vi "Begin.vi"(8 "error in":errorcluster) -> (0 "error out":errorcluster)   [LabVIEW 2018]
doc: "Called before other user functions, this VI is expected to open initial I/O refnums, load in file data, and do all program initialization. Notice that the <B>error out</B> terminal is simply used for data flow. Wiring it to other structures or subVIs ensures that this VI runs first."
uses:
  <vilib>/Rock Robotics/SystemInterfaces/DIO/FPGA_DIOPWMChannel.ctl
  <vilib>/Rock Robotics/WPI/SafetyOutput/WPI_SafetyOutputConfigMenu.ctl
  <vilib>/Rock Robotics/WPI/DriverStation/WPI_DriverStationRobotMode2.ctl
  <vilib>/Rock Robotics/WPI/Joystick/WPI_JoystickDeviceEnum.ctl
  <vilib>/Rock Robotics/SystemInterfaces/AI/FPGA_AIChannel.ctl
  <vilib>/Rock Robotics/WPI/RobotDrive/WPI_RobotDriveOpen2MotorWithTalon.vi
  Robot Global Data.vi
  <vilib>/Rock Robotics/Network Tables/NT Write String Array.vi
  <vilib>/Rock Robotics/WPI/ThirdParty/Phoenix-LabVIEW/Pigeon IMU/CTRE_PigeonIMU_Open_TalonSRX.vi
  <vilib>/Rock Robotics/WPI/Solenoid/WPI_SolenoidOpenSingle.vi
panel:
  in  "error in 2":errorcluster
  out "error out 2":errorcluster
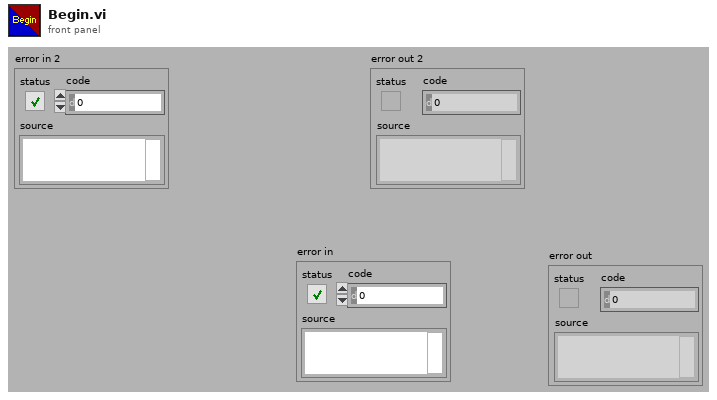
[diagram p1: front panel]
types:
  T1 = typedef "FPGA_AIChannel.ctl" = enum8{"AI 0", "AI 1", "AI 2", "AI 3", "AI MXP 0", "AI MXP 1", "AI MXP 2", "AI MXP 3", "Invalid"}
  T2 = typedef "WPI_JoystickDeviceEnum.ctl" = enum16{"USB 0", "USB 1", "USB 2", "USB 3", "USB 4", "USB 5"}
  T3 = typedef "WPI_DriverStationRobotMode2.ctl" = enum16{"Autonomous Disabled", "Autonomous Enabled", "Teleop Disabled", "Teleop Enabled", "Disconnected", "Finish", "Test Disabled", "Test Enabled", "Emergency Stopped"}
  T4 = typedef "WPI_SafetyOutputConfigMenu.ctl" = enum16{"Enable", "Disable"}
  T5 = typedef "FPGA_DIOPWMChannel.ctl" = enum8{"PWM 0", "PWM 1", "PWM 2", "PWM 3", "PWM 4", "PWM 5", "PWM 6", "PWM 7", "PWM 8", "PWM 9", "PWM MXP 0", "PWM MXP 1", "PWM MXP 2", "PWM MXP 3", "PWM MXP 4", "PWM MXP 5", "PWM MXP 6", "PWM MXP 7", "PWM MXP 8", "PWM MXP 9", "Invalid"}
  T6 = typedef "WPI_JoystickDevRef.ctl" = cluster{"Device":T2}
  T7 = typedef "WPI_RobotDriveDevRef.ctl" = cluster{"DevStatus":errorcluster, "Motors[]":T8[], "Square Inputs":bool, "Max Output":dbl}
  T8 = typedef "WPI_MotorControlDeviceRef.ctl" = cluster{"DeviceStatus":errorcluster, "Type":T9, "PWM":cluster{"PWM Channel":T5, "DeadBand":T10}, "CAN":cluster{"Device Number":u8, "SetOutput VI Ref":variant, "GetOutput VI Ref":variant, "Enable VI Ref":variant, "Disable VI Ref":variant, "Data":variant}, "Invert":bool, "DIO PWM":cluster{"PWM \"Enable\" Channel":T5, "DIOChannel":T11, "PWM Rate":dbl}}
  T9 = typedef "WPI_MotorControlType.ctl" = enum16{"PWM", "CAN", "DIO PWM"}
  T10 = typedef "WPI_PWMDeadband.ctl" = cluster{"Name":string, "maxPositivePwm":i32, "minPositivePwm":i32, "centerPwm":i32, "maxNegativePwm":i32, "minNegativePwm":i32, "angularRange":u16}
  T11 = typedef "FPGA_DIOChannel.ctl" = enum8{"DIO 0", "DIO 1", "DIO 2", "DIO 3", "DIO 4", "DIO 5", "DIO 6", "DIO 7", "DIO 8", "DIO 9", "DIO MXP 0", "DIO MXP 1", "DIO MXP 2", "DIO MXP 3", "DIO MXP 4", "DIO MXP 5", "DIO MXP 6", "DIO MXP 7", "DIO MXP 8", "DIO MXP 9", "DIO MXP 10", "DIO MXP 11", "DIO MXP 12", "DIO MXP 13", "DIO MXP 14", "DIO MXP 15", "SPI Port CS1", "SPI Port CS2", "SPI Port CS3", "SPI Port MISO", "SPI Port MOSI", "Invalid"}
  T12 = typedef "WPI_AnalogChannelDevRef.ctl" = cluster{"DevStatus":errorcluster, "Analog Channel":T1}
  T13 = typedef "CTRE_PigeonIMU_DeviceRef.ctl" = cluster{"DeviceStatus":errorcluster, "Device Number":u8, "Type":T14, "Device ID":u32, "Handle":u64, "UsageFrame":u32, "Library Path":path}
  T14 = typedef "CTRE_PigeonIMU_ConnectionType.ctl" = u32
  T15 = typedef "WPI_SolenoidDevRef.ctl" = cluster{"DevStatus":errorcluster, "Pneumatics Control Module":u8, "Forward Solenoid Channel":T16, "Reverse Solenoid Channel":T16}
  T16 = typedef "WPI_SolenoidChannel.ctl" = enum8{"Solenoid 0", "Solenoid 1", "Solenoid 2", "Solenoid 3", "Solenoid 4", "Solenoid 5", "Solenoid 6", "Solenoid 7", "Invalid"}
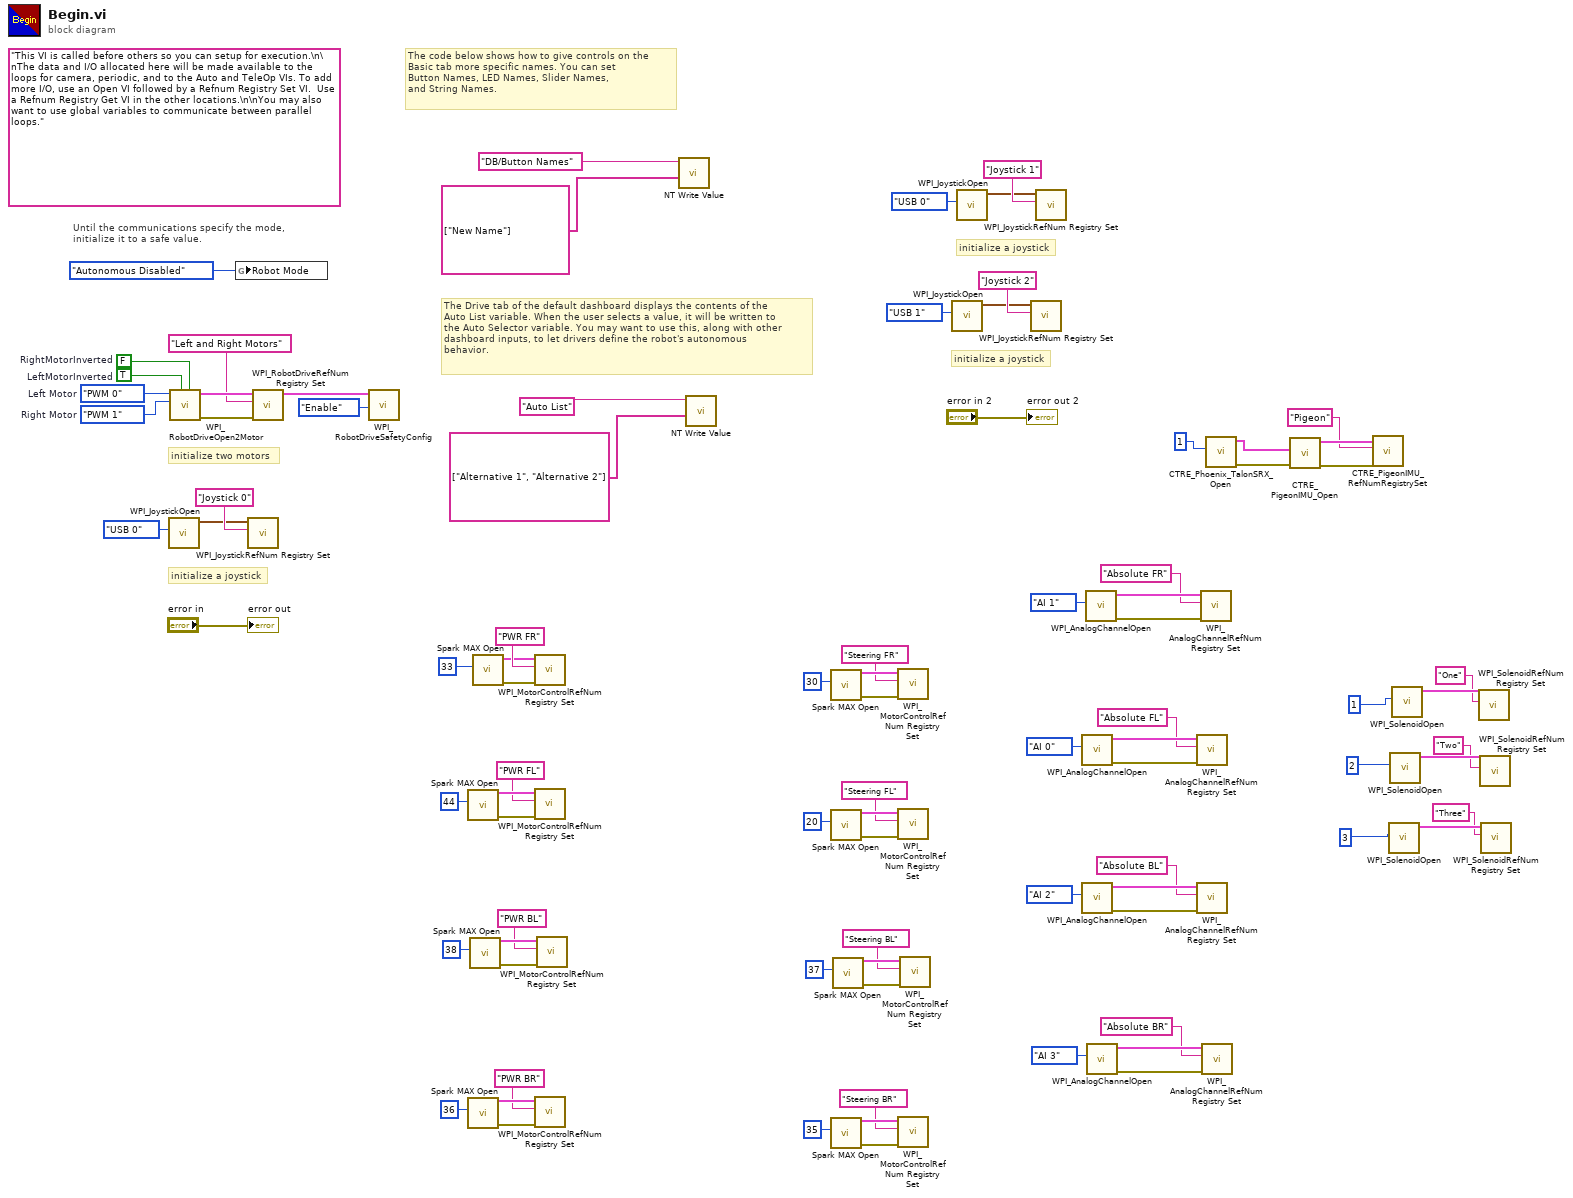
[diagram p0: block diagram]
diagram:
  (unwired) "This VI is called before others so you can setup for execution.\n\nThe data and I/O allocated here will be made available to the loops for camera, periodic, and to the Auto and TeleOp VIs. To add more I/O, use an Open VI followed by a Refnum Registry Set VI.  Use a Refnum Registry Get VI in the other locations.\n\nYou may also want to use global variables to communicate between parallel loops."
  w82 = FPGA_DIOPWMChannel."PWM 1"  # Right Motor
  w83 = FPGA_DIOPWMChannel."PWM 0"  # Left Motor
  w87 = TRUE  # LeftMotorInverted
  w88 = FALSE  # RightMotorInverted
  # "initialize a joystick"
  # "The Drive tab of the default dashboard displays the contents of the\nAuto List variable. When the user selects a value, it will be written to\nthe Auto Selector variable. You may want to use this, along with other\ndashboard inputs, to let drivers define the robot's autonomous\nbehavior."
  # "The code below shows how to give controls on the\nBasic tab more specific names. You can set\nButton Names, LED Names, Slider Names,\nand String Names."
  # "initialize a joystick"
  # "initialize a joystick"
  # "Until the communications specify the mode,\ninitialize it to a safe value."
  # "initialize two motors"
  n1 = call <vilib>:"WPI_JoystickOpen.vi"("JoystickDevice"=WPI_JoystickDeviceEnum."USB 0") -> ("JoystickDevRef"=w77:T6)  [unwired: 10 in]
  n2 = call-poly <vilib>:"WPI_RobotDriveOpen2Motor.vi"("Right Motor Inverted"=w88, "Left Motor Inverted"=w87, "Right Motor"=w82, "Left Motor"=w83) -> ("error out"=w84:errorcluster, "RobotDriveDevRef"=w86:T7)  [unwired: 1 in, 5 out]
  n3 = global write "Robot Global Data.vi" "Robot Mode"(WPI_DriverStationRobotMode2."Autonomous Disabled" ("Robot Mode")) -> ()
  n4 = call <vilib>:"WPI_JoystickRefNum Registry Set.vi"("refnum name"="Joystick 0", "JoystickDevRef"=w77) -> ()  [unwired: 8 in, 2 out]
  n5 = call <vilib>:"WPI_RobotDriveRefNum Registry Set.vi"("error in (no error)"=w84, "refnum name"="Left and Right Motors", "RobotDriveDevRef"=w86) -> ("RobotDriveDevRef"=w81:T7)  [unwired: 1 in, 7 out]
  n6 = call <vilib>:"WPI_RobotDriveSafetyConfig.vi"("mode"=WPI_SafetyOutputConfigMenu."Enable", "RobotDriveDevRef"=w81) -> ()  [unwired: 8 in, 2 out]
  n7 = call <vilib>:"Spark MAX Open.vi"("Device Number"=u8 44) -> ("error out"=w61:errorcluster, "MotorControlDeviceRef"=w62:T8)  [unwired: 9 in]
  n8 = call <vilib>:"Spark MAX Open.vi"("Device Number"=u8 36) -> ("error out"=w55:errorcluster, "MotorControlDeviceRef"=w56:T8)  [unwired: 9 in]
  n9 = call <vilib>:"Spark MAX Open.vi"("Device Number"=u8 38) -> ("error out"=w58:errorcluster, "MotorControlDeviceRef"=w59:T8)  [unwired: 9 in]
  n10 = call <vilib>:"Spark MAX Open.vi"("Device Number"=u8 33) -> ("error out"=w52:errorcluster, "MotorControlDeviceRef"=w53:T8)  [unwired: 9 in]
  n11 = call <vilib>:"WPI_MotorControlRefNum Registry Set.vi"("error in (no error)"=w52, "refnum name"="PWR FR", "MotorControlDevRef"=w53) -> ()  [unwired: 7 in, 2 out]
  n12 = call <vilib>:"WPI_MotorControlRefNum Registry Set.vi"("error in (no error)"=w61, "refnum name"="PWR FL", "MotorControlDevRef"=w62) -> ()  [unwired: 7 in, 2 out]
  n13 = call <vilib>:"WPI_MotorControlRefNum Registry Set.vi"("error in (no error)"=w55, "refnum name"="PWR BR", "MotorControlDevRef"=w56) -> ()  [unwired: 7 in, 2 out]
  n14 = call <vilib>:"WPI_MotorControlRefNum Registry Set.vi"("error in (no error)"=w58, "refnum name"="PWR BL", "MotorControlDevRef"=w59) -> ()  [unwired: 7 in, 2 out]
  n15 = call-poly <vilib>:"NT Write Value.vi"("String Array"=string[] ["New Name"], "Name"="DB/Button Names") -> ()  [unwired: 9 in, 1 out]
  n16 = call-poly <vilib>:"NT Write Value.vi"("String Array"=string[] ["Alternative 1", "Alternative 2"], "Name"="Auto List") -> ()  [unwired: 9 in, 1 out]
  n17 = call <vilib>:"Spark MAX Open.vi"("Device Number"=u8 30) -> ("error out"=w46:errorcluster, "MotorControlDeviceRef"=w47:T8)  [unwired: 9 in]
  n18 = call <vilib>:"Spark MAX Open.vi"("Device Number"=u8 20) -> ("error out"=w43:errorcluster, "MotorControlDeviceRef"=w44:T8)  [unwired: 9 in]
  n19 = call <vilib>:"Spark MAX Open.vi"("Device Number"=u8 35) -> ("error out"=w37:errorcluster, "MotorControlDeviceRef"=w38:T8)  [unwired: 9 in]
  n20 = call <vilib>:"Spark MAX Open.vi"("Device Number"=u8 37) -> ("error out"=w40:errorcluster, "MotorControlDeviceRef"=w41:T8)  [unwired: 9 in]
  n21 = call <vilib>:"WPI_MotorControlRefNum Registry Set.vi"("error in (no error)"=w46, "refnum name"="Steering FR", "MotorControlDevRef"=w47) -> ()  [unwired: 7 in, 2 out]
  n22 = call <vilib>:"WPI_MotorControlRefNum Registry Set.vi"("error in (no error)"=w43, "refnum name"="Steering FL", "MotorControlDevRef"=w44) -> ()  [unwired: 7 in, 2 out]
  n23 = call <vilib>:"WPI_MotorControlRefNum Registry Set.vi"("error in (no error)"=w37, "refnum name"="Steering BR", "MotorControlDevRef"=w38) -> ()  [unwired: 7 in, 2 out]
  n24 = call <vilib>:"WPI_MotorControlRefNum Registry Set.vi"("error in (no error)"=w40, "refnum name"="Steering BL", "MotorControlDevRef"=w41) -> ()  [unwired: 7 in, 2 out]
  n25 = call <vilib>:"WPI_JoystickOpen.vi"("JoystickDevice"=WPI_JoystickDeviceEnum."USB 1") -> ("JoystickDevRef"=w65:T6)  [unwired: 10 in]
  n26 = call <vilib>:"WPI_JoystickOpen.vi"("JoystickDevice"=WPI_JoystickDeviceEnum."USB 0") -> ("JoystickDevRef"=w73:T6)  [unwired: 10 in]
  n27 = call <vilib>:"WPI_JoystickRefNum Registry Set.vi"("refnum name"="Joystick 2", "JoystickDevRef"=w65) -> ()  [unwired: 8 in, 2 out]
  n28 = call <vilib>:"WPI_JoystickRefNum Registry Set.vi"("refnum name"="Joystick 1", "JoystickDevRef"=w73) -> ()  [unwired: 8 in, 2 out]
  n29 = call <vilib>:"WPI_AnalogChannelOpen.vi"("Analog Channel"=FPGA_AIChannel."AI 0") -> ("error out"=w28:errorcluster, "AIDeviceRef"=w27:T12)  [unwired: 9 in]
  n30 = call <vilib>:"WPI_AnalogChannelOpen.vi"("Analog Channel"=FPGA_AIChannel."AI 2") -> ("error out"=w25:errorcluster, "AIDeviceRef"=w24:T12)  [unwired: 9 in]
  n31 = call <vilib>:"WPI_AnalogChannelOpen.vi"("Analog Channel"=FPGA_AIChannel."AI 1") -> ("error out"=w31:errorcluster, "AIDeviceRef"=w30:T12)  [unwired: 9 in]
  n32 = call <vilib>:"WPI_AnalogChannelOpen.vi"("Analog Channel"=FPGA_AIChannel."AI 3") -> ("error out"=w22:errorcluster, "AIDeviceRef"=w21:T12)  [unwired: 9 in]
  n33 = call <vilib>:"WPI_AnalogChannelRefNum Registry Set.vi"("error in (no error)"=w28, "refnum name"="Absolute FL", "AIDeviceRef"=w27) -> ()  [unwired: 7 in, 2 out]
  n34 = call <vilib>:"WPI_AnalogChannelRefNum Registry Set.vi"("error in (no error)"=w25, "refnum name"="Absolute BL", "AIDeviceRef"=w24) -> ()  [unwired: 7 in, 2 out]
  n35 = call <vilib>:"WPI_AnalogChannelRefNum Registry Set.vi"("error in (no error)"=w31, "refnum name"="Absolute FR", "AIDeviceRef"=w30) -> ()  [unwired: 7 in, 2 out]
  n36 = call <vilib>:"WPI_AnalogChannelRefNum Registry Set.vi"("error in (no error)"=w22, "refnum name"="Absolute BR", "AIDeviceRef"=w21) -> ()  [unwired: 7 in, 2 out]
  n37 = call <vilib>:"CTRE_Phoenix_TalonSRX_Open.vi"("Device Number"=1) -> ("error out"=w11:errorcluster, "CAN Talon SRX Ref"=w12:T8)  [unwired: 9 in]
  n38 = call-poly <vilib>:"CTRE_PigeonIMU_Open.vi"("error in"=w11, "CAN Talon SRX Ref"=w12) -> ("error out"=w10:errorcluster, "PigeonIMUDevRef"=w15:T13)  [unwired: 8 in]
  n39 = call <vilib>:"CTRE_PigeonIMU_RefNumRegistrySet.vi"("error in (no error)"=w10, "refnum name"="Pigeon", "PigeonIMUDevRef"=w15) -> ()  [unwired: 7 in, 2 out]
  n40 = call-poly <vilib>:"WPI_SolenoidOpen.vi"("Solenoid Channel"=3) -> ("SolenoidDevRef"=w9:T15)  [unwired: 9 in, 1 out]
  n41 = call-poly <vilib>:"WPI_SolenoidOpen.vi"("Solenoid Channel"=2) -> ("SolenoidDevRef"=w8:T15)  [unwired: 9 in, 1 out]
  n42 = call-poly <vilib>:"WPI_SolenoidOpen.vi"("Solenoid Channel"=1) -> ("SolenoidDevRef"=w7:T15)  [unwired: 9 in, 1 out]
  n43 = call <vilib>:"WPI_SolenoidRefNum Registry Set.vi"("refnum name"="One", "SolenoidDevRef"=w7) -> ()  [unwired: 8 in, 2 out]
  n44 = call <vilib>:"WPI_SolenoidRefNum Registry Set.vi"("refnum name"="Two", "SolenoidDevRef"=w8) -> ()  [unwired: 8 in, 2 out]
  n45 = call <vilib>:"WPI_SolenoidRefNum Registry Set.vi"("refnum name"="Three", "SolenoidDevRef"=w9) -> ()  [unwired: 8 in, 2 out]
  "error out" <- "error in"
  "error out 2" <- "error in 2"
